vi "Project_References_Global.vi"() -> ()   [LabVIEW 2021]
panel:
  out "INI References":T1(array[cluster])
  out "CTL References":T1(array[cluster])
  out "Global References":T1(array[cluster])
  out "VI References":T1(array[cluster])
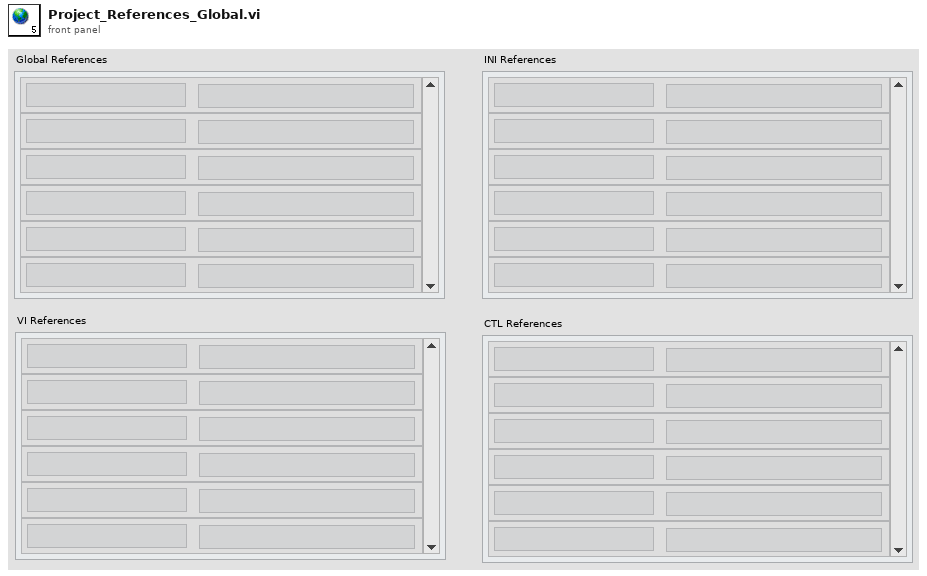
[diagram p1: front panel]
types:
  T1 = cluster{"VI Name":string, "String Path":string}[]
diagram:
